vi "set_filter_constant.vi"(8 "error in (no error)":errorcluster, 10 "Filter constant":string(combo)="0", 11 "VISA Refnum in":refnum<visa-resource-name>) -> (0 "error out":errorcluster, 3 "VISA Refnum out":refnum<visa-resource-name>)   [LabVIEW 2018]
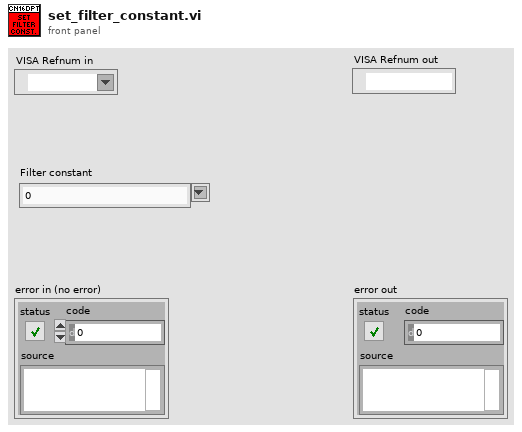
[diagram p1: front panel]
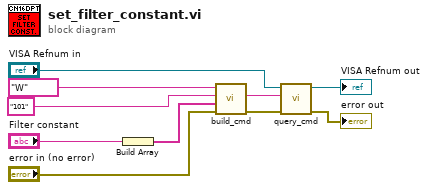
[diagram p0: block diagram]
diagram:
  n1 = Build Array("Filter constant") -> (w2:string[])
  n2 = call "build_cmd.vi"("error in (no error)"="error in (no error)", "Parameter list"=w2, "Command ID"="101", "Command class"="W") -> ("error out"=w5:errorcluster, "Command"=w4:string)  [unwired: 6 in]
  n3 = call "query_cmd.vi"("error in (no error)"=w5, "Command"=w4, "VISA resource name"="VISA Refnum in") -> ("error out"=→"error out":errorcluster, "VISA resource name out"=→"VISA Refnum out":refnum<visa-resource-name>)  [unwired: 6 in, 1 out]
